vi "Set Table.vi"(6 "Error In":errorcluster, 8 "Table":string[][](array[string])=[["50", "", "Start Fail"], ["02h", "", "Overload"], ["04h", "", "Under Speed (1550 rpm or lower)"], ["10h", "", "Short Circuit"], ["20h", "", "Over Temperature"], ["80h", "", "Set Speed Out of Range"], ["", "00h", "Compreessor Running"], ["", "FFh", "Compressor Stopped"]], 9 "Column Head":string[](array[string])=["Force(lbs)", "Name", "Description"]) -> (0 "Error Out":errorcluster, 3 "Select code":string[](array[string])=["02h", "", "Overload"])   [LabVIEW 2019]
panel:
  in  "Code Info":i32[](listbox)=[1]
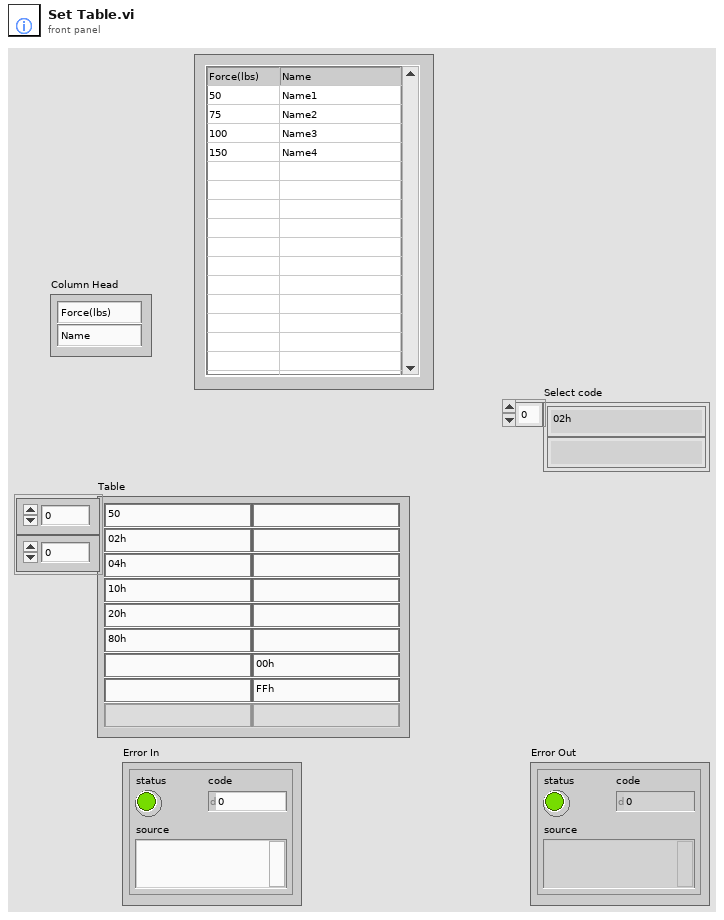
[diagram p1: front panel]
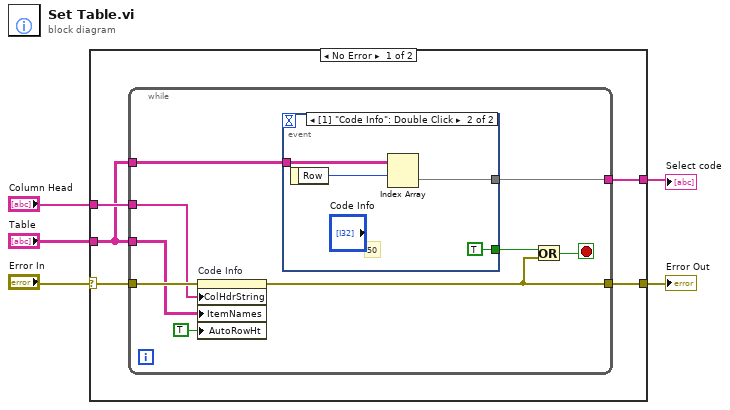
[diagram p0: block diagram]
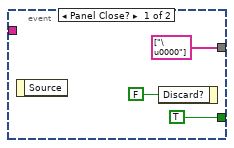
[diagram p2: hidden frame]
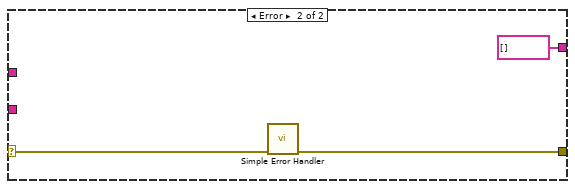
[diagram p3: hidden frame]
diagram:
  # "50"
  n1 = case shown="No Error" "Error In" {
    selector: "Error In" -> [w10 w29]
    tunnel: [w8 w28] -> w4
    tunnel: "Table" -> [w7 _]
    tunnel: "Column Head" -> [w9 _]
    tunnel: [w6 string[] [] ("Table")] -> w1
    frame No Error {
      n2 = while {
        tunnel: w10 -> [w18]
        tunnel: w7 -> [w12]
        tunnel: w9 -> [w13]
        tunnel: [w16] -> w8
        tunnel: w7 -> [w14]
        tunnel: [w11] -> w6
        stop <- w15 stop-if-true
        n3 = property on="Code Info" class="MCListbox (strict)"(error in=w18, "ColHdrString"=w13, "ItemNames"=w12, "AutoRowHt"=TRUE ("Autosizing Row Height")) -> (error out=w16:errorcluster)  [unwired: 1 in, 1 out]
        n4 = event shown="[1] \"Code Info\": Double Click" {
          selector: _ -> [_ _]
          dyn-events: _ -> [_ _]
          timeout: _ -> [_ _]
          tunnel: [TRUE ("Discard?") TRUE ("Discard?")] -> w17
          tunnel: w14 -> [_ w25]
          tunnel: [string[] ["\u0000"] ("Table") w24] -> w11
          event Panel Close? {
            n5 = event-data() -> ()  [unwired: 1 in, 1 out]
            n6 = event-data("Discard?"=FALSE) -> ()  [unwired: 1 in, 1 out]
          }
          event "Code Info": Double Click {
            n7 = event-data() -> ("Row"=w26:i32)  [unwired: 1 in]
            n8 = Index Array(array=w25, index (row)=w26) -> (element=w24:string[])  [unwired: 1 in]
          }
        }
        n9 = Or(x=w17, y=w16) -> (x .or. y?=w15:bool)
      }
    }
    frame Error {
      n10 = call <vilib>:"Simple Error Handler.vi"("error in (no error)"=w29) -> ("error out"=w28:errorcluster)  [unwired: 4 in, 4 out]
    }
  }
  "Error Out" <- w4
  "Select code" <- w1
